vi "Angle_change.vi"(11 "in":dbl) -> (3 "out":dbl)   [LabVIEW 2014]
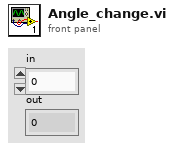
[diagram p1: front panel]
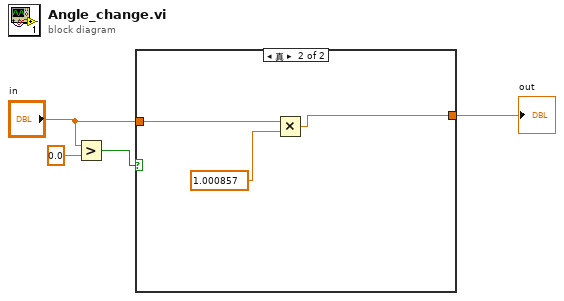
[diagram p0: block diagram]
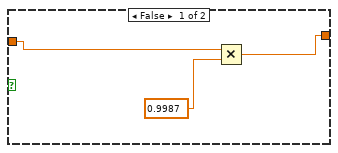
[diagram p2: hidden frame]
diagram:
  n1 = Greater?(x="in", y=0.0) -> (0:w3:bool)
  n2 = case shown="真" w3 {
    tunnel: "in" -> [w5 w10]
    tunnel: [w6 w9] -> w1
    frame False {
      n3 = Multiply(x=w5, y=0.9987) -> (x*y=w6:dbl)
    }
    frame True {
      n4 = Multiply(x=w10, y=1.000857) -> (x*y=w9:dbl)
    }
  }
  "out" <- w1
